vi "HCC Board ID Configuration.vi"(0 "Station and Board IDs":path, 5 "Error In":errorcluster) -> (8 "Agilent Channels DAQ":string="213,214,215,216,217,218,219,220", 10 "all rows":string[][](array[string])=[["Agilent Alias", "AGILENT236", ""], ["Current Transducer Type", " 1", ""], ["2M1", "", ""], ["2M2", "", ""], ["2M3", "", ""], ["2M4", "", ""], ["2M5", "", ""], ["2M6", "", ""], ["2M7", "", ""], ["2M8", "", ""], ["2M9", "", ""], ["2M10", "", ""], ["2M11", "", ""], ["2M12", "", ""], ["2M13", "7200002F", "213"], ["2M14", "72000040", "214"], ["2M15", "72000036", "215"], ["2M16", "7200003F", "216"], ["2M17", "7200003E", "217"], ["2M18", "72000387", "218"], ["2M19", "7200002E", "219"], ["2M20", "72000035", "220"], ["N/A", "", ""], ["N/A", "", ""], ["N/A", "", ""], ["N/A", "", ""]], 11 "Disable Channel = True":bool[](array[boolean])=[TRUE, TRUE, TRUE, TRUE, TRUE, TRUE, TRUE, TRUE, TRUE, TRUE, TRUE, TRUE, FALSE, FALSE, FALSE, FALSE, FALSE, FALSE, FALSE, FALSE, TRUE, TRUE, TRUE, TRUE], 14 "34972A_1":refnum<visa-resource-name>, 15 "34972A_2":refnum<visa-resource-name>, 16 "Station IDs":string[](array[string])=["2M1", "2M2", "2M3", "2M4", "2M5", "2M6", "2M7", "2M8", "2M9", "2M10", "2M11", "2M12", "2M13", "2M14", "2M15", "2M16", "2M17", "2M18", "2M19", "2M20", "N/A", "N/A", "N/A", "N/A"], 17 "Board ID's":string[](array[string])=["", "", "", "", "", "", "", "", "", "", "", "", "7200002F", "72000040", "72000036", "7200003F", "7200003E", "72000387", "7200002E", "72000035", "", "", "", ""], 18 "Voltage Indexes":i32[](array[numeric]), 19 "Error Out":errorcluster)   [LabVIEW 2016]
uses:
  <vilib>/Utility/file.llb/Read Delimited Spreadsheet (string).vi
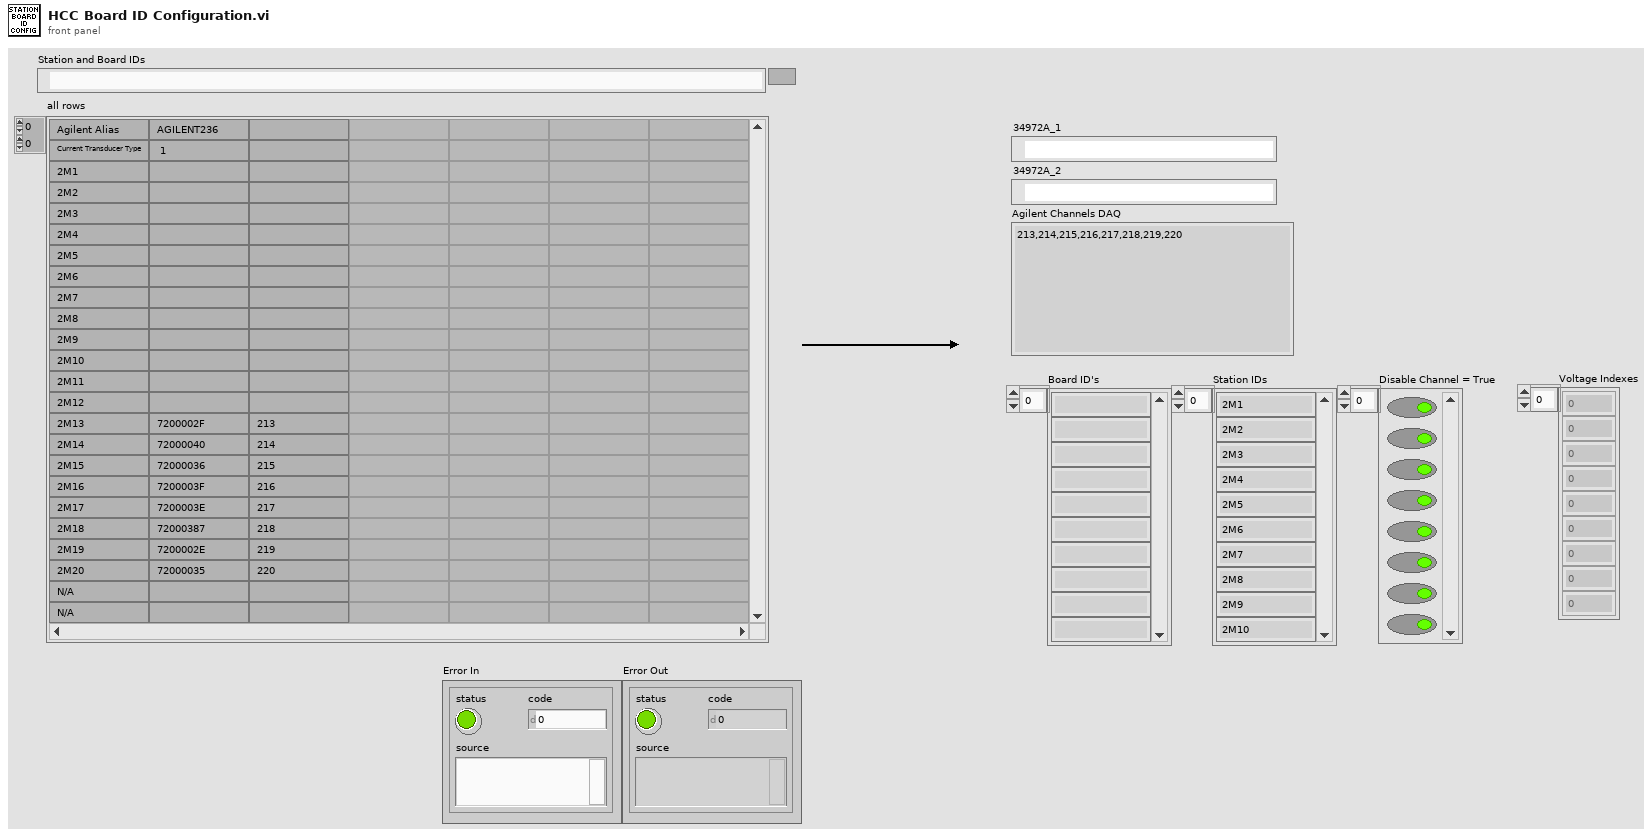
[diagram p1: front panel]
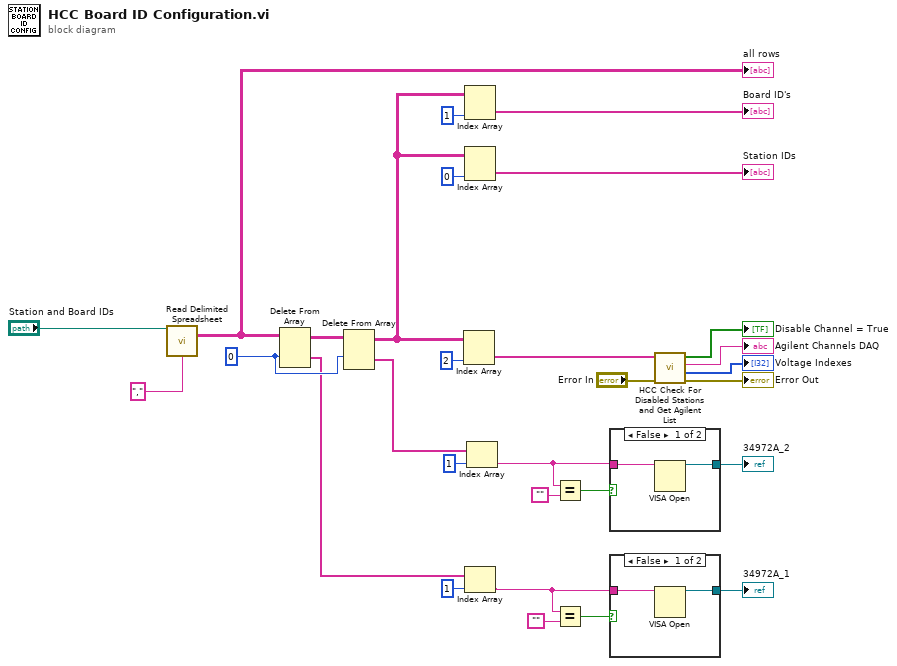
[diagram p0: block diagram]
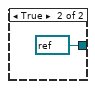
[diagram p2: hidden frame]
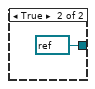
[diagram p3: hidden frame]
diagram:
  w17 = 0 ("index (row)")
  n1 = call-poly <vilib>:"Read Delimited Spreadsheet.vi"("file path (dialog if empty)"="Station and Board IDs", "delimiter (\\t)"="," ("delimiter (\\t)")) -> ("all rows"=w1:string[][])  [unwired: 8 in, 5 out]
  "all rows" <- w1
  n2 = Delete From Array(array=w1, index (row)=w17) -> (deleted portion=w11:string[], array with subset deleted=w21:string[][])  [unwired: 2 in]
  n3 = Delete From Array(array=w21, index (row)=w17) -> (deleted portion=w19:string[], array with subset deleted=w20:string[][])  [unwired: 2 in]
  n4 = Index Array(array=w20, index (col)=2 ("disabled index (col)")) -> (element=w16:string[])  [unwired: 1 in]
  n5 = Index Array(array=w20, index (col)=1 ("disabled index (col)")) -> (element=→"Board ID's":string[])  [unwired: 1 in]
  n6 = Index Array(array=w20, index (col)=0 ("disabled index (col)")) -> (element=→"Station IDs":string[])  [unwired: 1 in]
  n7 = Index Array(array=w11, index=1) -> (element=w4:string)
  n8 = Index Array(array=w19, index=1) -> (element=w7:string)
  n9 = Equal?(x=w7, y="") -> (x = y?=w8:bool)
  n10 = Equal?(x=w4, y="") -> (x = y?=w6:bool)
  n11 = case shown="False" w8 {
    tunnel: [w31 refnum<visa-resource-name> refnum ("VISA resource name")] -> w10
    tunnel: w7 -> [w30 _]
    frame False {
      n12 = VISA Open(VISA resource name=w30) -> (VISA resource name=w31:refnum<visa-resource-name>)  [unwired: 4 in, 1 out]
    }
    frame True {
    }
  }
  "34972A_2" <- w10
  n13 = case shown="False" w6 {
    tunnel: [w34 refnum<visa-resource-name> refnum ("VISA resource name")] -> w3
    tunnel: w4 -> [w33 _]
    frame False {
      n14 = VISA Open(VISA resource name=w33) -> (VISA resource name=w34:refnum<visa-resource-name>)  [unwired: 4 in, 1 out]
    }
    frame True {
    }
  }
  "34972A_1" <- w3
  n15 = call "HCC Check For Disabled Stations and Get Agilent List.vi"("Error In"="Error In", "Agilent Channels"=w16) -> ("Error Out"=→"Error Out":errorcluster, "Voltage Indexes"=→"Voltage Indexes":i32[], "Agilent Channels DAQ"=→"Agilent Channels DAQ":string, "Disable Channel = True"=→"Disable Channel = True":bool[])  [unwired: 6 in]
